vi "Sensor Close.vi"   [LabVIEW 2014]
types:
  T1 = typedef "WPI_PotentiometerDevRef.ctl" = cluster{"DevStatus":errorcluster, "Controller":T2, "Analog Channel":T3, "Invert Output":bool}
  T2 = typedef "FPGA_TypedefAnalogModule.ctl" = enum16{"Controller 1"}
  T3 = typedef "FPGA_AIChannel.ctl" = enum8{"AI 0", "AI 1", "AI 2", "AI 3", "AI MXP 0", "AI MXP 1", "AI MXP 2", "AI MXP 3", "Invalid"}
  T4 = typedef "WPI_SwitchDevRef.ctl" = cluster{"DevStatus":errorcluster, "DIO Channel":T5, "Controller":T6, "CntIndex":T7, "Normally Closed":bool}
  T5 = typedef "FPGA_DIOChannel.ctl" = enum8{"DIO 0", "DIO 1", "DIO 2", "DIO 3", "DIO 4", "DIO 5", "DIO 6", "DIO 7", "DIO 8", "DIO 9", "DIO MXP 0", "DIO MXP 1", "DIO MXP 2", "DIO MXP 3", "DIO MXP 4", "DIO MXP 5", "DIO MXP 6", "DIO MXP 7", "DIO MXP 8", "DIO MXP 9", "DIO MXP 10", "DIO MXP 11", "DIO MXP 12", "DIO MXP 13", "DIO MXP 14", "DIO MXP 15", "Invalid"}
  T6 = typedef "FPGA_TypedefDigitalModule.ctl" = enum16{"Controller 1"}
  T7 = typedef "FPGA_CounterCtrSystemIndex.ctl" = enum8{"Ctr 0", "Ctr 1", "Ctr 2", "Ctr 3", "Ctr 4", "Ctr 5", "Ctr 6", "Ctr 7", "Invalid"}
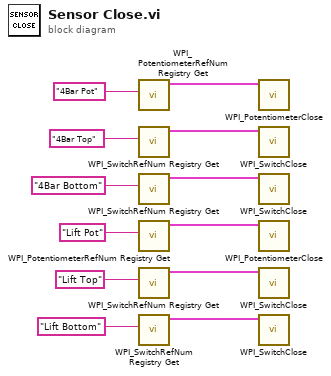
[diagram p0: block diagram]
diagram:
  n1 = call <vilib>:"WPI_PotentiometerRefNum Registry Get.vi"("refnum name"="4Bar Pot") -> ("PotDevRef"=w12:T1)  [unwired: 9 in, 1 out]
  n2 = call <vilib>:"WPI_SwitchRefNum Registry Get.vi"("refnum name"="4Bar Top") -> ("SwitchDevRef"=w11:T4)  [unwired: 9 in, 1 out]
  n3 = call <vilib>:"WPI_SwitchRefNum Registry Get.vi"("refnum name"="4Bar Bottom") -> ("SwitchDevRef"=w10:T4)  [unwired: 9 in, 1 out]
  n4 = call <vilib>:"WPI_PotentiometerRefNum Registry Get.vi"("refnum name"="Lift Pot") -> ("PotDevRef"=w6:T1)  [unwired: 9 in, 1 out]
  n5 = call <vilib>:"WPI_SwitchRefNum Registry Get.vi"("refnum name"="Lift Top") -> ("SwitchDevRef"=w4:T4)  [unwired: 9 in, 1 out]
  n6 = call <vilib>:"WPI_SwitchRefNum Registry Get.vi"("refnum name"="Lift Bottom") -> ("SwitchDevRef"=w2:T4)  [unwired: 9 in, 1 out]
  n7 = call <vilib>:"WPI_PotentiometerClose.vi"("PotDevRef"=w12) -> ()  [unwired: 10 in, 1 out]
  n8 = call <vilib>:"WPI_SwitchClose.vi"("SwitchDevRef"=w11) -> ()  [unwired: 10 in, 1 out]
  n9 = call <vilib>:"WPI_SwitchClose.vi"("SwitchDevRef"=w10) -> ()  [unwired: 10 in, 1 out]
  n10 = call <vilib>:"WPI_PotentiometerClose.vi"("PotDevRef"=w6) -> ()  [unwired: 10 in, 1 out]
  n11 = call <vilib>:"WPI_SwitchClose.vi"("SwitchDevRef"=w4) -> ()  [unwired: 10 in, 1 out]
  n12 = call <vilib>:"WPI_SwitchClose.vi"("SwitchDevRef"=w2) -> ()  [unwired: 10 in, 1 out]
